vi "RunAction.vi"(8 "ErrorIn":errorcluster, 9 "Timeout (s)":dbl, 10 "Action":string, 11 "TopModuleIn":refnum<class "TopModule.lvclass">) -> (0 "ErrorOut":errorcluster, 1 "Timeout?":bool, 3 "TopModuleOut":refnum<class "TopModule.lvclass">)   [LabVIEW 2019, in "TopModule.lvclass"]
uses:
  TopModule.lvclass
  TopModule.lvclass/TopModule.ctl
  IAction/IAction.lvclass
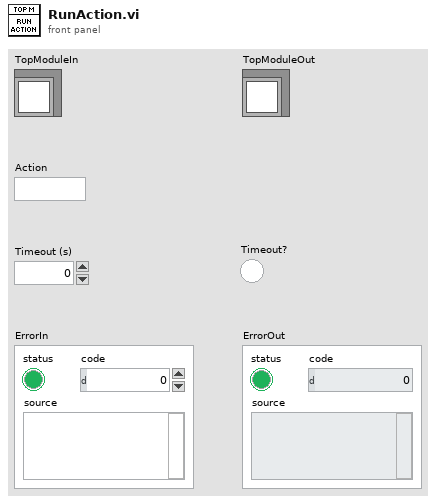
[diagram p1: front panel]
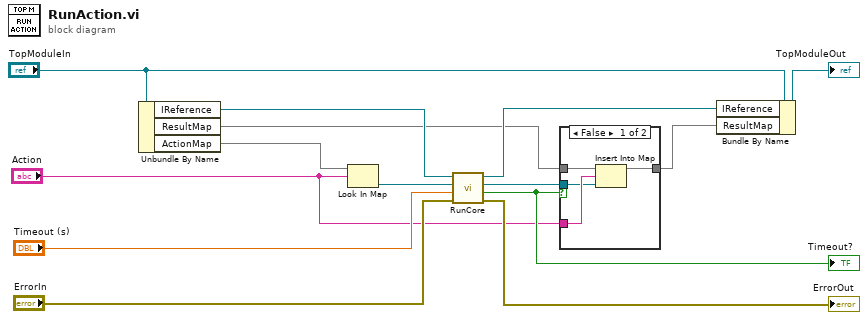
[diagram p0: block diagram]
diagram:
  n1 = Unbundle By Name("TopModuleIn") -> ("IReference"=w7:refnum<class "IReference.lvclass">, "ResultMap"=w6:map{string, refnum<class "IResult.lvclass">}, "ActionMap"=w12:map{string, refnum<class "IAction.lvclass">})
  n2 = Look In Map(map=w12, key="Action") -> (value=w11:refnum<class "IAction.lvclass">)  [unwired: 1 in, 1 out]
  n3 = call-dynamic "RunCore.vi"("Error In"="ErrorIn", "Timeout (s)"="Timeout (s)", "MeasIn"=w11, "HardwareIn"=w7) -> ("Error Out"=→"ErrorOut":errorcluster, "Timeout?"=w2:bool, "ResultOut"=w4:refnum<class "IResult.lvclass">, "HardwareOut"=w8:refnum<class "IReference.lvclass">)  [unwired: 4 in]
  "Timeout?" <- w2
  n4 = case shown="False" w2 {
    tunnel: "Action" -> [w18 _]
    tunnel: w6 -> [w17 w19]
    tunnel: [w16 w19] -> w5
    tunnel: w4 -> [w15 _]
    frame False {
      n5 = Insert Into Map(map in=w17, key=w18, value=w15) -> (map out=w16:map{string, refnum<class "IResult.lvclass">})  [unwired: 2 out]
    }
    frame True {
    }
  }
  n6 = Bundle By Name(cluster="TopModuleIn", "IReference"=w8, "ResultMap"=w5) -> (→"TopModuleOut":refnum<class "TopModule.lvclass">)
